vi "rsidr_core_global.vi"() -> ()   [LabVIEW 2015, in "Rohde&Schwarz CMXP GPRF.lvlib"] (continued)
Callback"="", "Supported Models"="", "Instrument Options"="", "Flags"=0, "Help"="Returns the traces of the spectrum diagram. The current, average, minimum and maximum traces can be retrieved.\nEach trace contains 801 power values and covers the configured frequency span.\n\nAvailable Repeated Capabilities:\ninstance: i0, i1, i2, i3, i4, i5, i6, i7, i8, i9, i10, i11, i12, i13, i14, i15, i16, i17, i18, i19, i20, i21, i22, i23, i24, i25, i26, i27, i28, i29, i30, i31, i32\r\n\nRemote-control command(s):\nFETCh:GPRF:MEAS<i>:FFTSanalyzer:POWer:MINimum?"}, {"Level"=3, "Class Only"=FALSE, "Identifier"="RSCMXPGPRF_ATTR_FETCH_FFT_MEASUREMENT_POWER_MAXIMUM", "Descriptive Name"="Fetch FFT Measurement Power Maximum", "Data Type"=6, "Command"="FETC:GPRF:MEAS{instance}:FFTS:POW:MAX?", "Access"=0, "Range Table"="", "Read Callback"="", "Write Callback"="", "Supported Models"="", "Instrument Options"="", "Flags"=0, "Help"="Returns the traces of the spectrum diagram. The current, average, minimum and maximum traces can be retrieved.\nEach trace contains 801 power values and covers the configured frequency span.\n\nAvailable Repeated Capabilities:\ninstance: i0, i1, i2, i3, i4, i5, i6, i7, i8, i9, i10, i11, i12, i13, i14, i15, i16, i17, i18, i19, i20, i21, i22, i23, i24, i25, i26, i27, i28, i29, i30, i31, i32\r\n\nRemote-control command(s):\nFETCh:GPRF:MEAS<i>:FFTSanalyzer:POWer:MAXimum?"}, {"Level"=3, "Class Only"=FALSE, "Identifier"="RSCMXPGPRF_ATTR_READ_FFT_MEASUREMENT_PEAK_SEARCH_RESULT_CURRENT", "Descriptive Name"="Read FFT Measurement Peak Search Result Current", "Data Type"=6, "Command"="READ:GPRF:MEAS{instance}:FFTS:PEAK:CURR?", "Access"=0, "Range Table"="", "Read Callback"="", "Write Callback"="", "Supported Models"="", "Instrument Options"="", "Flags"=0, "Help"="Returns the results of the peak search in the spectrum diagram. Separate commands retrieve results for the current trace and for the average trace.\nThe results are returned in the following order:\n<Reliability>, {<Frequency>, <Level>}marker 0, ..., {<Frequency>, <Level>}marker 4\n\nAvailable Repeated Capabilities:\ninstance: i0, i1, i2, i3, i4, i5, i6, i7, i8, i9, i10, i11, i12, i13, i14, i15, i16, i17, i18, i19, i20, i21, i22, i23, i24, i25, i26, i27, i28, i29, i30, i31, i32\r\n\nRemote-control command(s):\nREAD:GPRF:MEAS<i>:FFTSanalyzer:PEAKs:CURRent?"}, {"Level"=3, "Class Only"=FALSE, "Identifier"="RSCMXPGPRF_ATTR_READ_FFT_MEASUREMENT_PEAK_SEARCH_RESULT_AVERAGE", "Descriptive Name"="Read FFT Measurement Peak Search Result Average", "Data Type"=6, "Command"="READ:GPRF:MEAS{instance}:FFTS:PEAK:AVER?", "Access"=0, "Range Table"="", "Read Callback"="", "Write Callback"="", "Supported Models"="", "Instrument Options"="", "Flags"=0, "Help"="Returns the results of the peak search in the spectrum diagram. Separate commands retrieve results for the current trace and for the average trace.\nThe results are returned in the following order:\n<Reliability>, {<Frequency>, <Level>}marker 0, ..., {<Frequency>, <Level>}marker 4\n\nAvailable Repeated Capabilities:\ninstance: i0, i1, i2, i3, i4, i5, i6, i7, i8, i9, i10, i11, i12, i13, i14, i15, i16, i17, i18, i19, i20, i21, i22, i23, i24, i25, i26, i27, i28, i29, i30, i31, i32\r\n\nRemote-control command(s):\nREAD:GPRF:MEAS<i>:FFTSanalyzer:PEAKs:AVERage?"}, {"Level"=3, "Class Only"=FALSE, "Identifier"="RSCMXPGPRF_ATTR_FETCH_FFT_MEASUREMENT_PEAK_SEARCH_RESULT_CURRENT", "Descriptive Name"="Fetch FFT Measurement Peak Search Result Current", "Data Type"=6, "Command"="FETC:GPRF:MEAS{instance}:FFTS:PEAK:CURR?", "Access"=0, "Range Table"="", "Read Callback"="", "Write Callback"="", "Supported Models"="", "Instrument Options"="", "Flags"=0, "Help"="Returns the results of the peak search in the spectrum diagram. Separate commands retrieve results for the current trace and for the average trace.\nThe results are returned in the following order:\n<Reliability>, {<Frequency>, <Level>}marker 0, ..., {<Frequency>, <Level>}marker 4\n\nAvailable Repeated Capabilities:\ninstance: i0, i1, i2, i3, i4, i5, i6, i7, i8, i9, i10, i11, i12, i13, i14, i15, i16, i17, i18, i19, i20, i21, i22, i23, i24, i25, i26, i27, i28, i29, i30, i31, i32\r\n\nRemote-control command(s):\nFETCh:GPRF:MEAS<i>:FFTSanalyzer:PEAKs:CURRent?"}, {"Level"=3, "Class Only"=FALSE, "Identifier"="RSCMXPGPRF_ATTR_FETCH_FFT_MEASUREMENT_PEAK_SEARCH_RESULT_AVERAGE", "Descriptive Name"="Fetch FFT Measurement Peak Search Result Average", "Data Type"=6, "Command"="FETC:GPRF:MEAS{instance}:FFTS:PEAK:AVER?", "Access"=0, "Range Table"="", "Read Callback"="", "Write Callback"="", "Supported Models"="", "Instrument Options"="", "Flags"=0, "Help"="Returns the results of the peak search in the spectrum diagram. Separate commands retrieve results for the current trace and for the average trace.\nThe results are returned in the following order:\n<Reliability>, {<Frequency>, <Level>}marker 0, ..., {<Frequency>, <Level>}marker 4\n\nAvailable Repeated Capabilities:\ninstance: i0, i1, i2, i3, i4, i5, i6, i7, i8, i9, i10, i11, i12, i13, i14, i15, i16, i17, i18, i19, i20, i21, i22, i23, i24, i25, i26, i27, i28, i29, i30, i31, i32\r\n\nRemote-control command(s):\nFETCh:GPRF:MEAS<i>:FFTSanalyzer:PEAKs:AVERage?"}, {"Level"=3, "Class Only"=FALSE, "Identifier"="RSCMXPGPRF_ATTR_READ_FFT_MEASUREMENT_IQ_AMPLITUDES_I", "Descriptive Name"="Read FFT Measurement IQ Amplitudes I", "Data Type"=6, "Command"="READ:GPRF:MEAS{instance}:FFTS:I?", "Access"=0, "Range Table"="", "Read Callback"="", "Write Callback"="", "Supported Models"="", "Instrument Options"="", "Flags"=0, "Help"="Returns the measured normalized I and Q amplitudes in the time domain.\n\nAvailable Repeated Capabilities:\ninstance: i0, i1, i2, i3, i4, i5, i6, i7, i8, i9, i10, i11, i12, i13, i14, i15, i16, i17, i18, i19, i20, i21, i22, i23, i24, i25, i26, i27, i28, i29, i30, i31, i32\r\n\nRemote-control command(s):\nREAD:GPRF:MEAS<i>:FFTSanalyzer:I?"}, {"Level"=3, "Class Only"=FALSE, "Identifier"="RSCMXPGPRF_ATTR_READ_FFT_MEASUREMENT_IQ_AMPLITUDES_Q", "Descriptive Name"="Read FFT Measurement IQ Amplitudes Q", "Data Type"=6, "Command"="READ:GPRF:MEAS{instance}:FFTS:Q?", "Access"=0, "Range Table"="", "Read Callback"="", "Write Callback"="", "Supported Models"="", "Instrument Options"="", "Flags"=0, "Help"="Returns the measured normalized I and Q amplitudes in the time domain.\n\nAvailable Repeated Capabilities:\ninstance: i0, i1, i2, i3, i4, i5, i6, i7, i8, i9, i10, i11, i12, i13, i14, i15, i16, i17, i18, i19, i20, i21, i22, i23, i24, i25, i26, i27, i28, i29, i30, i31, i32\r\n\nRemote-control command(s):\nREAD:GPRF:MEAS<i>:FFTSanalyzer:Q?"}, {"Level"=3, "Class Only"=FALSE, "Identifier"="RSCMXPGPRF_ATTR_FETCH_FFT_MEASUREMENT_IQ_AMPLITUDES_I", "Descriptive Name"="Fetch FFT Measurement IQ Amplitudes I", "Data Type"=6, "Command"="FETC:GPRF:MEAS{instance}:FFTS:I?", "Access"=0, "Range Table"="", "Read Callback"="", "Write Callback"="", "Supported Models"="", "Instrument Options"="", "Flags"=0, "Help"="Returns the measured normalized I and Q amplitudes in the time domain.\n\nAvailable Repeated Capabilities:\ninstance: i0, i1, i2, i3, i4, i5, i6, i7, i8, i9, i10, i11, i12, i13, i14, i15, i16, i17, i18, i19, i20, i21, i22, i23, i24, i25, i26, i27, i28, i29, i30, i31, i32\r\n\nRemote-control command(s):\nFETCh:GPRF:MEAS<i>:FFTSanalyzer:I?"}, {"Level"=3, "Class Only"=FALSE, "Identifier"="RSCMXPGPRF_ATTR_FETCH_FFT_MEASUREMENT_IQ_AMPLITUDES_Q", "Descriptive Name"="Fetch FFT Measurement IQ Amplitudes Q", "Data Type"=6, "Command"="FETC:GPRF:MEAS{instance}:FFTS:Q?", "Access"=0, "Range Table"="", "Read Callback"="", "Write Callback"="", "Supported Models"="", "Instrument Options"="", "Flags"=0, "Help"="Returns the measured normalized I and Q amplitudes in the time domain.\n\nAvailable Repeated Capabilities:\ninstance: i0, i1, i2, i3, i4, i5, i6, i7, i8, i9, i10, i11, i12, i13, i14, i15, i16, i17, i18, i19, i20, i21, i22, i23, i24, i25, i26, i27, i28, i29, i30, i31, i32\r\n\nRemote-control command(s):\nFETCh:GPRF:MEAS<i>:FFTSanalyzer:Q?"}, {"Level"=1, "Class Only"=TRUE, "Identifier"="", "Descriptive Name"="Capture Analyzer", "Data Type"=0, "Command"="", "Access"=0, "Range Table"="", "Read Callback"="", "Write Callback"="", "Supported Models"="", "Instrument Options"="", "Flags"=0, "Help"="Configures the Capture Analyzer Square."}, {"Level"=2, "Class Only"=TRUE, "Identifier"="", "Descriptive Name"="Configuration", "Data Type"=0, "Command"="", "Access"=0, "Range Table"="", "Read Callback"="", "Write Callback"="", "Supported Models"="", "Instrument Options"="", "Flags"=0, "Help"="Configures the Capture Analyzer Square."}, {"Level"=3, "Class Only"=FALSE, "Identifier"="RSCMXPGPRF_ATTR_CAPTURE_ANALYZER_MEASUREMENT_SEGMENT", "Descriptive Name"="Capture Analyzer Measurement Segment", "Data Type"=0, "Command"="CONF:GPRF:MEAS{instance}:CAN:SEGM", "Access"=2, "Range Table"="", "Read Callback"="", "Write Callback"="", "Supported Models"="", "Instrument Options"="", "Flags"=0, "Help"="Selects a segment of a list mode measurement for result analysis.\nThe selection affects the GUI contents and the contents stored by the command CONFigure:GPRF:MEAS<i>:CANalyzer:IQFile.\n\nAvailable Repeated Capabilities:\ninstance: i0, i1, i2, i3, i4, i5, i6, i7, i8, i9, i10, i11, i12, i13, i14, i15, i16, i17, i18, i19, i20, i21, i22, i23, i24, i25, i26, i27, i28, i29, i30, i31, i32\r\n\nRemote-control command(s):\nCONFigure:GPRF:MEAS<i>:CANalyzer:SEGMent"}, {"Level"=3, "Class Only"=FALSE, "Identifier"="RSCMXPGPRF_ATTR_CAPTURE_ANALYZER_MEASUREMENT_STEP", "Descriptive Name"="Capture Analyzer Measurement Step", "Data Type"=0, "Command"="CONF:GPRF:MEAS{instance}:CAN:STEP", "Access"=2, "Range Table"="", "Read Callback"="", "Write Callback"="", "Supported Models"="", "Instrument Options"="", "Flags"=0, "Help"="Selects a step of a list mode measurement for result analysis.\nThe selection affects the GUI contents and the contents stored by the command CONFigure:GPRF:MEAS<i>:CANalyzer:IQFile.\n\nAvailable Repeated Capabilities:\ninstance: i0, i1, i2, i3, i4, i5, i6, i7, i8, i9, i10, i11, i12, i13, i14, i15, i16, i17, i18, i19, i20, i21, i22, i23, i24, i25, i26, i27, i28, i29, i30, i31, i32\r\n\nRemote-control command(s):\nCONFigure:GPRF:MEAS<i>:CANalyzer:STEP"}, {"Level"=3, "Class Only"=FALSE, "Identifier"="RSCMXPGPRF_ATTR_CAPTURE_ANALYZER_MEASUREMENT_SAVE_IQ_FILE", "Descriptive Name"="Capture Analyzer Measurement Save IQ File", "Data Type"=2, "Command"="CONF:GPRF:MEAS{instance}:CAN:IQF", "Access"=2, "Range Table"="", "Read Callback"="", "Write Callback"="", "Supported Models"="", "Instrument Options"="", "Flags"=0, "Help"="Saves the I/Q data for the current step to the selected file.\n\nAvailable Repeated Capabilities:\ninstance: i0, i1, i2, i3, i4, i5, i6, i7, i8, i9, i10, i11, i12, i13, i14, i15, i16, i17, i18, i19, i20, i21, i22, i23, i24, i25, i26, i27, i28, i29, i30, i31, i32\r\n\nRemote-control command(s):\nCONFigure:GPRF:MEAS<i>:CANalyzer:IQFile"}, {"Level"=3, "Class Only"=FALSE, "Identifier"="RSCMXPGPRF_ATTR_CAPTURE_ANALYZER_MEASUREMENT_STORAGE_FOLDER", "Descriptive Name"="Capture Analyzer Measurement Storage Folder", "Data Type"=2, "Command"="CONF:GPRF:MEAS{instance}:CAN:SALL:IQF", "Access"=2, "Range Table"="", "Read Callback"="", "Write Callback"="", "Supported Models"="", "Instrument Options"="", "Flags"=0, "Help"="Selects a folder for storage of all buffer contents to files (I/Q data for all segments).\nThe default folder is @USERDATA\\captureanalyzer. You can only select a subfolder of this default folder.\nAll files within the selected folder are deleted when the capture buffer analyzer writes the result files.\n\nAvailable Repeated Capabilities:\ninstance: i0, i1, i2, i3, i4, i5, i6, i7, i8, i9, i10, i11, i12, i13, i14, i15, i16, i17, i18, i19, i20, i21, i22, i23, i24, i25, i26, i27, i28, i29, i30, i31, i32\r\n\nRemote-control command(s):\nCONFigure:GPRF:MEAS<i>:CANalyzer:SALL:IQFolder"}, {"Level"=3, "Class Only"=FALSE, "Identifier"="RSCMXPGPRF_ATTR_CAPTURE_ANALYZER_MEASUREMENT_WRITE_TO_FILE", "Descriptive Name"="Capture Analyzer Measurement Write to File", "Data Type"=3, "Command"="CONF:GPRF:MEAS{instance}:CAN:SALL:WTF", "Access"=2, "Range Table"="", "Read Callback"="", "Write Callback"="", "Supported Models"="", "Instrument Options"="", "Flags"=0, "Help"="Enables or disables saving of all buffer contents to files (I/Q data for all segments).\nWith <WriteToFolder> = ON, the files are stored when the capture buffer analyzer is started.\n\nAvailable Repeated Capabilities:\ninstance: i0, i1, i2, i3, i4, i5, i6, i7, i8, i9, i10, i11, i12, i13, i14, i15, i16, i17, i18, i19, i20, i21, i22, i23, i24, i25, i26, i27, i28, i29, i30, i31, i32\r\n\nRemote-control command(s):\nCONFigure:GPRF:MEAS<i>:CANalyzer:SALL:WTFolder"}, {"Level"=2, "Class Only"=TRUE, "Identifier"="", "Descriptive Name"="Control", "Data Type"=0, "Command"="", "Access"=0, "Range Table"="", "Read Callback"="", "Write Callback"="", "Supported Models"="", "Instrument Options"="", "Flags"=0, "Help"="Configures the Capture Analyzer Square Control."}, {"Level"=3, "Class Only"=FALSE, "Identifier"="RSCMXPGPRF_ATTR_CAPTURE_ANALYZER_MEASUREMENT_INIT", "Descriptive Name"="Capture Analyzer Measurement Init", "Data Type"=4, "Command"="INIT:GPRF:MEAS{instance}:CAN", "Access"=1, "Range Table"="", "Read Callback"="", "Write Callback"="", "Supported Models"="", "Instrument Options"="", "Flags"=0, "Help"="Starts the measurement.\n\nAvailable Repeated Capabilities:\ninstance: i0, i1, i2, i3, i4, i5, i6, i7, i8, i9, i10, i11, i12, i13, i14, i15, i16, i17, i18, i19, i20, i21, i22, i23, i24, i25, i26, i27, i28, i29, i30, i31, i32\r\n\nRemote-control command(s):\nINITiate:GPRF:MEAS<i>:CANalyzer"}, {"Level"=3, "Class Only"=FALSE, "Identifier"="RSCMXPGPRF_ATTR_CAPTURE_ANALYZER_MEASUREMENT_ABORT", "Descriptive Name"="Capture Analyzer Measurement Abort", "Data Type"=4, "Command"="ABOR:GPRF:MEAS{instance}:CAN", "Access"=1, "Range Table"="", "Read Callback"="", "Write Callback"="", "Supported Models"="", "Instrument Options"="", "Flags"=0, "Help"="Aborts the measurement.\n\nAvailable Repeated Capabilities:\ninstance: i0, i1, i2, i3, i4, i5, i6, i7, i8, i9, i10, i11, i12, i13, i14, i15, i16, i17, i18, i19, i20, i21, i22, i23, i24, i25, i26, i27, i28, i29, i30, i31, i32\r\n\nRemote-control command(s):\nABORt:GPRF:MEAS<i>:CANalyzer"}, {"Level"=3, "Class Only"=FALSE, "Identifier"="RSCMXPGPRF_ATTR_CAPTURE_ANALYZER_MEASUREMENT_STOP", "Descriptive Name"="Capture Analyzer Measurement Stop", "Data Type"=4, "Command"="STOP:GPRF:MEAS{instance}:CAN", "Access"=1, "Range Table"="", "Read Callback"="", "Write Callback"="", "Supported Models"="", "Instrument Options"="", "Flags"=0, "Help"="Stops the measurement.\n\nAvailable Repeated Capabilities:\ninstance: i0, i1, i2, i3, i4, i5, i6, i7, i8, i9, i10, i11, i12, i13, i14, i15, i16, i17, i18, i19, i20, i21, i22, i23, i24, i25, i26, i27, i28, i29, i30, i31, i32\r\n\nRemote-control command(s):\nSTOP:GPRF:MEAS<i>:CANalyzer"}, {"Level"=3, "Class Only"=FALSE, "Identifier"="RSCMXPGPRF_ATTR_CAPTURE_ANALYZER_MEASUREMENT_STATUS", "Descriptive Name"="Capture Analyzer Measurement Status", "Data Type"=6, "Command"="FETC:GPRF:MEAS{instance}:CAN:STAT?", "Access"=0, "Range Table"="", "Read Callback"="", "Write Callback"="", "Supported Models"="", "Instrument Options"="", "Flags"=0, "Help"="Queries the main measurement state.\n\nAvailable Repeated Capabilities:\ninstance: i0, i1, i2, i3, i4, i5, i6, i7, i8, i9, i10, i11, i12, i13, i14, i15, i16, i17, i18, i19, i20, i21, i22, i23, i24, i25, i26, i27, i28, i29, i30, i31, i32\r\n\nRemote-control command(s):\nFETCh:GPRF:MEAS<i>:CANalyzer:STATe?"}, {"Level"=3, "Class Only"=FALSE, "Identifier"="RSCMXPGPRF_ATTR_CAPTURE_ANALYZER_MEASUREMENT_STATUS_ALL", "Descriptive Name"="Capture Analyzer Measurement Status All", "Data Type"=6, "Command"="FETC:GPRF:MEAS{instance}:CAN:STAT:ALL?", "Access"=0, "Range Table"="", "Read Callback"="", "Write Callback"="", "Supported Models"="", "Instrument Options"="", "Flags"=0, "Help"="Queries the main measurement state and the measurement substates. Both measurement substates are relevant for running measurements only.\n\nAvailable Repeated Capabilities:\ninstance: i0, i1, i2, i3, i4, i5, i6, i7, i8, i9, i10, i11, i12, i13, i14, i15, i16, i17, i18, i19, i20, i21, i22, i23, i24, i25, i26, i27, i28, i29, i30, i31, i32\r\n\nRemote-control command(s):\nFETCh:GPRF:MEAS<i>:CANalyzer:STATe:ALL?"}, {"Level"=3, "Class Only"=FALSE, "Identifier"="RSCMXPGPRF_ATTR_CAPTURE_ANALYZER_MEASUREMENT_FIRMWARE", "Descriptive Name"="Capture Analyzer Measurement Firmware", "Data Type"=2, "Command"="CONF:GPRF:MEAS{instance}:CAN:MNAM?", "Access"=0, "Range Table"="", "Read Callback"="", "Write Callback"="", "Supported Models"="", "Instrument Options"="", "Flags"=0, "Help"="Queries which firmware application has captured the data.\n\nAvailable Repeated Capabilities:\ninstance: i0, i1, i2, i3, i4, i5, i6, i7, i8, i9, i10, i11, i12, i13, i14, i15, i16, i17, i18, i19, i20, i21, i22, i23, i24, i25, i26, i27, i28, i29, i30, i31, i32\r\n\nRemote-control command(s):\nCONFigure:GPRF:MEAS<i>:CANalyzer:MNAMe?"}, {"Level"=1, "Class Only"=TRUE, "Identifier"="", "Descriptive Name"="NRPM", "Data Type"=0, "Command"="", "Access"=0, "Range Table"="", "Read Callback"="", "Write Callback"="", "Supported Models"="", "Instrument Options"="", "Flags"=0, "Help"="Configures the NRPM Square."}, {"Level"=2, "Class Only"=TRUE, "Identifier"="", "Descriptive Name"="Configuration", "Data Type"=0, "Command"="", "Access"=0, "Range Table"="", "Read Callback"="", "Write Callback"="", "Supported Models"="", "Instrument Options"="", "Flags"=0, "Help"="Configures the NRPM Square."}, {"Level"=3, "Class Only"=FALSE, "Identifier"="RSCMXPGPRF_ATTR_NRPM_MEASUREMENT_FREQUENCY", "Descriptive Name"="NRPM Measurement Frequency", "Data Type"=1, "Command"="CONF:GPRF:MEAS{instance}:NRPM:SENS{sensor}:FREQ", "Access"=2, "Range Table"="rsCmxpGprf_rngNRPMMeasurementFrequency", "Read Callback"="", "Write Callback"="", "Supported Models"="", "Instrument Options"="", "Flags"=0, "Help"="Specifies the input frequency at the power sensor connected to Sensor.\n\nAvailable Repeated Capabilities:\ninstance: i0, i1, i2, i3, i4, i5, i6, i7, i8, i9, i10, i11, i12, i13, i14, i15, i16, i17, i18, i19, i20, i21, i22, i23, i24, i25, i26, i27, i28, i29, i30, i31, i32\r\nsensor: sensor1, sensor2, sensor3\r\n\nRemote-control command(s):\nCONFigure:GPRF:MEAS<i>:NRPM:SENSor<no>:FREQuency"}, {"Level"=3, "Class Only"=FALSE, "Identifier"="RSCMXPGPRF_ATTR_NRPM_MEASUREMENT_TIMEOUT", "Descriptive Name"="NRPM Measurement Timeout", "Data Type"=1, "Command"="CONF:GPRF:MEAS{instance}:NRPM:TOUT", "Access"=2, "Range Table"="", "Read Callback"="", "Write Callback"="", "Supported Models"="", "Instrument Options"="", "Flags"=0, "Help"="Defines a timeout for the measurement. The timer is started when the measurement is initiated via a READ or INIT command. It is not started if the measurement is initiated manually ([ON | OFF] key or [RESTART | STOP] key).When the measurement has completed the first measurement cycle (first single shot), the statistical depth is reached and the timer is reset.If the first measurement cycle has not been completed when the timer expires, the measurement is stopped. The measurement state  changes to RDY. The reliability indicator is set to 1, indicating that a measurement timeout occurred. Still running READ, FETCh or CALCulate commands are completed, returning the available results. At least for some results, there are no values at all or the statistical depth has not been reached.A timeout of 0 s corresponds to an infinite measurement timeout.\n\nAvailable Repeated Capabilities:\ninstance: i0, i1, i2, i3, i4, i5, i6, i7, i8, i9, i10, i11, i12, i13, i14, i15, i16, i17, i18, i19, i20, i21, i22, i23, i24, i25, i26, i27, i28, i29, i30, i31, i32\r\n\nRemote-control command(s):\nCONFigure:GPRF:MEAS<i>:NRPM:TOUT"}, {"Level"=3, "Class Only"=FALSE, "Identifier"="RSCMXPGPRF_ATTR_NRPM_MEASUREMENT_STATISTIC_COUNT", "Descriptive Name"="NRPM Measurement Statistic Count", "Data Type"=0, "Command"="CONF:GPRF:MEAS{instance}:NRPM:SCO", "Access"=2, "Range Table"="rsCmxpGprf_rngNRPMStatCount", "Read Callback"="", "Write Callback"="", "Supported Models"="", "Instrument Options"="", "Flags"=0, "Help"="Specifies the statistic count of the measurement. The statistic count is equal to the number of measurement intervals per single shot.\n\nAvailable Repeated Capabilities:\ninstance: i0, i1, i2, i3, i4, i5, i6, i7, i8, i9, i10, i11, i12, i13, i14, i15, i16, i17, i18, i19, i20, i21, i22, i23, i24, i25, i26, i27, i28, i29, i30, i31, i32\r\n\nRemote-control command(s):\nCONFigure:GPRF:MEAS<i>:NRPM:SCOunt"}, {"Level"=3, "Class Only"=FALSE, "Identifier"="RSCMXPGPRF_ATTR_NRPM_MEASUREMENT_REPETITION", "Descriptive Name"="NRPM Measurement Repetition", "Data Type"=0, "Command"="CONF:GPRF:MEAS{instance}:NRPM:REP", "Access"=2, "Range Table"="rsCmxpGprf_rngRepMode", "Read Callback"="", "Write Callback"="", "Supported Models"="", "Instrument Options"="", "Flags"=0, "Help"="Specifies the repetition mode of the measurement. The repetition mode specifies whether the measurement is stopped after a single shot or repeated continuously. Use CONFigure:..:MEAS<i>:...:SCOunt to determine the number of measurement intervals per single shot.\n\nAvailable Repeated Capabilities:\ninstance: i0, i1, i2, i3, i4, i5, i6, i7, i8, i9, i10, i11, i12, i13, i14, i15, i16, i17, i18, i19, i20, i21, i22, i23, i24, i25, i26, i27, i28, i29, i30, i31, i32\r\n\nRemote-control command(s):\nCONFigure:GPRF:MEAS<i>:NRPM:REPetition"}, {"Level"=2, "Class Only"=TRUE, "Identifier"="", "Descriptive Name"="Control", "Data Type"=0, "Command"="", "Access"=0, "Range Table"="", "Read Callback"="", "Write Callback"="", "Supported Models"="", "Instrument Options"="", "Flags"=0, "Help"="Configures the NRPM Square Control."}, {"Level"=3, "Class Only"=FALSE, "Identifier"="RSCMXPGPRF_ATTR_NRPM_MEASUREMENT_INIT", "Descriptive Name"="NRPM Measurement Init", "Data Type"=4, "Command"="INIT:GPRF:MEAS{instance}:NRPM", "Access"=1, "Range Table"="", "Read Callback"="", "Write Callback"="", "Supported Models"="", "Instrument Options"="", "Flags"=0, "Help"="Starts the measurement.\n\nAvailable Repeated Capabilities:\ninstance: i0, i1, i2, i3, i4, i5, i6, i7, i8, i9, i10, i11, i12, i13, i14, i15, i16, i17, i18, i19, i20, i21, i22, i23, i24, i25, i26, i27, i28, i29, i30, i31, i32\r\n\nRemote-control command(s):\nINITiate:GPRF:MEAS<i>:NRPM"}, {"Level"=3, "Class Only"=FALSE, "Identifier"="RSCMXPGPRF_ATTR_NRPM_MEASUREMENT_ABORT", "Descriptive Name"="NRPM Measurement Abort", "Data Type"=4, "Command"="ABOR:GPRF:MEAS{instance}:NRPM", "Access"=1, "Range Table"="", "Read Callback"="", "Write Callback"="", "Supported Models"="", "Instrument Options"="", "Flags"=0, "Help"="Aborts the measurement.\n\nAvailable Repeated Capabilities:\ninstance: i0, i1, i2, i3, i4, i5, i6, i7, i8, i9, i10, i11, i12, i13, i14, i15, i16, i17, i18, i19, i20, i21, i22, i23, i24, i25, i26, i27, i28, i29, i30, i31, i32\r\n\nRemote-control command(s):\nABORt:GPRF:MEAS<i>:NRPM"}, {"Level"=3, "Class Only"=FALSE, "Identifier"="RSCMXPGPRF_ATTR_NRPM_MEASUREMENT_STOP", "Descriptive Name"="NRPM Measurement Stop", "Data Type"=4, "Command"="STOP:GPRF:MEAS{instance}:NRPM", "Access"=1, "Range Table"="", "Read Callback"="", "Write Callback"="", "Supported Models"="", "Instrument Options"="", "Flags"=0, "Help"="Stops the measurement.\n\nAvailable Repeated Capabilities:\ninstance: i0, i1, i2, i3, i4, i5, i6, i7, i8, i9, i10, i11, i12, i13, i14, i15, i16, i17, i18, i19, i20, i21, i22, i23, i24, i25, i26, i27, i28, i29, i30, i31, i32\r\n\nRemote-control command(s):\nSTOP:GPRF:MEAS<i>:NRPM"}, {"Level"=3, "Class Only"=FALSE, "Identifier"="RSCMXPGPRF_ATTR_NRPM_MEASUREMENT_STATUS", "Descriptive Name"="NRPM Measurement Status", "Data Type"=6, "Command"="FETC:GPRF:MEAS{instance}:NRPM:STAT?", "Access"=0, "Range Table"="", "Read Callback"="", "Write Callback"="", "Supported Models"="", "Instrument Options"="", "Flags"=0, "Help"="Queries the main measurement state.\n\nAvailable Repeated Capabilities:\ninstance: i0, i1, i2, i3, i4, i5, i6, i7, i8, i9, i10, i11, i12, i13, i14, i15, i16, i17, i18, i19, i20, i21, i22, i23, i24, i25, i26, i27, i28, i29, i30, i31, i32\r\n\nRemote-control command(s):\nFETCh:GPRF:MEAS<i>:NRPM:STATe?"}, {"Level"=3, "Class Only"=FALSE, "Identifier"="RSCMXPGPRF_ATTR_NRPM_MEASUREMENT_STATUS_ALL", "Descriptive Name"="NRPM Measurement Status All", "Data Type"=6, "Command"="FETC:GPRF:MEAS{instance}:NRPM:STAT:ALL?", "Access"=0, "Range Table"="", "Read Callback"="", "Write Callback"="", "Supported Models"="", "Instrument Options"="", "Flags"=0, "Help"="Queries the main measurement state and the measurement substates. Both measurement substates are relevant for running measurements only.\n\nAvailable Repeated Capabilities:\ninstance: i0, i1, i2, i3, i4, i5, i6, i7, i8, i9, i10, i11, i12, i13, i14, i15, i16, i17, i18, i19, i20, i21, i22, i23, i24, i25, i26, i27, i28, i29, i30, i31, i32\r\n\nRemote-control command(s):\nFETCh:GPRF:MEAS<i>:NRPM:STATe:ALL?"}, {"Level"=2, "Class Only"=TRUE, "Identifier"="", "Descriptive Name"="Results", "Data Type"=0, "Command"="", "Access"=0, "Range Table"="", "Read Callback"="", "Write Callback"="", "Supported Models"="", "Instrument Options"="", "Flags"=0, "Help"="Queries the NRPM Square Results."}, {"Level"=3, "Class Only"=FALSE, "Identifier"="RSCMXPGPRF_ATTR_NRPM_MEASUREMENT_SENSOR_POWER", "Descriptive Name"="NRPM Measurement Sensor Power", "Data Type"=6, "Command"="CALC:GPRF:MEAS{instance}:NRPM:SENS{sensor}:POW?", "Access"=0, "Range Table"="", "Read Callback"="", "Write Callback"="", "Supported Models"="", "Instrument Options"="", "Flags"=0, "Help"="Returns the measurement results for the power sensor connected to Sensor <no>.\n\nAvailable Repeated Capabilities:\ninstance: i0, i1, i2, i3, i4, i5, i6, i7, i8, i9, i10, i11, i12, i13, i14, i15, i16, i17, i18, i19, i20, i21, i22, i23, i24, i25, i26, i27, i28, i29, i30, i31, i32\r\nsensor: sensor1, sensor2, sensor3\r\n\nRemote-control command(s):\nCALCulate:GPRF:MEAS<i>:NRPM:SENSor<no>:POWer?"}, {"Level"=3, "Class Only"=FALSE, "Identifier"="RSCMXPGPRF_ATTR_FETCH_NRPM_MEASUREMENT_SENSOR_POWER", "Descriptive Name"="Fetch NRPM Measurement Sensor Power", "Data Type"=6, "Command"="FETC:GPRF:MEAS{instance}:NRPM:SENS{sensor}:POW?", "Access"=0, "Range Table"="", "Read Callback"="", "Write Callback"="", "Supported Models"="", "Instrument Options"="", "Flags"=0, "Help"="Returns the measurement results for the power sensor connected to Sensor <no>.\n\nAvailable Repeated Capabilities:\ninstance: i0, i1, i2, i3, i4, i5, i6, i7, i8, i9, i10, i11, i12, i13, i14, i15, i16, i17, i18, i19, i20, i21, i22, i23, i24, i25, i26, i27, i28, i29, i30, i31, i32\r\nsensor: sensor1, sensor2, sensor3\r\n\nRemote-control command(s):\nFETCh:GPRF:MEAS<i>:NRPM:SENSor<no>:POWer?"}, {"Level"=3, "Class Only"=FALSE, "Identifier"="RSCMXPGPRF_ATTR_READ_NRPM_MEASUREMENT_SENSOR_POWER", "Descriptive Name"="Read NRPM Measurement Sensor Power", "Data Type"=6, "Command"="READ:GPRF:MEAS{instance}:NRPM:SENS{sensor}:POW?", "Access"=0, "Range Table"="", "Read Callback"="", "Write Callback"="", "Supported Models"="", "Instrument Options"="", "Flags"=0, "Help"="Returns the measurement results for the power sensor connected to Sensor <no>.\n\nAvailable Repeated Capabilities:\ninstance: i0, i1, i2, i3, i4, i5, i6, i7, i8, i9, i10, i11, i12, i13, i14, i15, i16, i17, i18, i19, i20, i21, i22, i23, i24, i25, i26, i27, i28, i29, i30, i31, i32\r\nsensor: sensor1, sensor2, sensor3\r\n\nRemote-control command(s):\nREAD:GPRF:MEAS<i>:NRPM:SENSor<no>:POWer?"}, {"Level"=1, "Class Only"=TRUE, "Identifier"="", "Descriptive Name"="Utility", "Data Type"=0, "Command"="", "Access"=0, "Range Table"="", "Read Callback"="", "Write Callback"="", "Supported Models"="", "Instrument Options"="", "Flags"=0, "Help"="Put a help here"}, {"Level"=2, "Class Only"=FALSE, "Identifier"="RSCMXPGPRF_ATTR_SYSTEM_VERSION", "Descriptive Name"="System Version", "Data Type"=2, "Command"="SYST:VERSion?", "Access"=0, "Range Table"="", "Read Callback"="", "Write Callback"="", "Supported Models"="", "Instrument Options"="", "Flags"=0, "Help"="Gets system version.\n\nAvailable Repeated Capabilities:\nNone\n\nRemote-control command(s):\nSYSTem:VERSion?"}, {"Level"=2, "Class Only"=FALSE, "Identifier"="RSCMXPGPRF_ATTR_SYSTEM_ERROR", "Descriptive Name"="System Error", "Data Type"=2, "Command"="SYST:ERRor?", "Access"=0, "Range Table"="", "Read Callback"="", "Write Callback"="", "Supported Models"="", "Instrument Options"="", "Flags"=0, "Help"="This attribute queries the earliest entry in the error queue, and deletes it after the readout.\n\nAvailable Repeated Capabilities:\nNone\n\nRemote-control command(s):\nSYSTem:ERRor?"}, {"Level"=2, "Class Only"=FALSE, "Identifier"="RSCMXPGPRF_ATTR_SYSTEM_ALL_ERRORS", "Descriptive Name"="System All Errors", "Data Type"=2, "Command"="SYST:ERR:ALL?", "Access"=0, "Range Table"="", "Read Callback"="", "Write Callback"="", "Supported Models"="", "Instrument Options"="", "Flags"=0, "Help"="Reads all errors from instrument.\n\nAvailable Repeated Capabilities:\nNone\n\nRemote-control command(s):\nSYSTem:ERRor:ALL?"}, {"Level"=2, "Class Only"=FALSE, "Identifier"="RSCMXPGPRF_ATTR_SYSTEM_PRESET", "Descriptive Name"="System Preset", "Data Type"=4, "Command"="SYST:PRES", "Access"=1, "Range Table"="", "Read Callback"="", "Write Callback"="", "Supported Models"="", "Instrument Options"="", "Flags"=0, "Help"="Resets instrument.\n\nAvailable Repeated Capabilities:\nNone\n\nRemote-control command(s):\nSYSTem:PRESet"}] {"Flags" format="%08b"; "Access" items=["Read Only", "Write Only", "Read/Write"]; "Data Type" items=["Integer 32", "Double", "String", "Boolean", "None", "Integer 64", "RawString"]}
  in  "Supported Models":string[](array[string])=["CMX", "CMP", "CMW"]
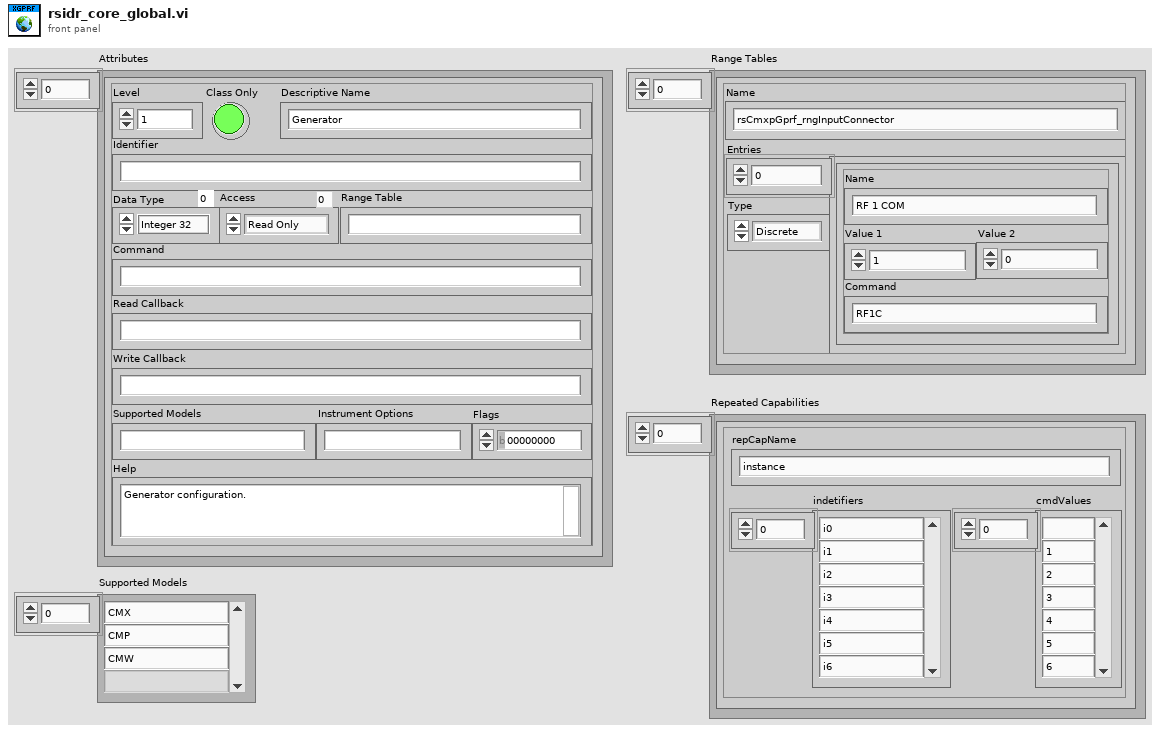
[diagram p1: front panel]
types:
  T1 = typedef "Rohde&Schwarz CMXP GPRF.lvlib/rsidr_core.lvlib/type_Input_Format_RepCap.ctl" = cluster{"repCapName":string, "indetifiers":string[], "cmdValues":string[]}
  T2 = typedef "Rohde&Schwarz CMXP GPRF.lvlib/rsidr_core.lvlib/type_Input_Format_RangeTable.ctl" = cluster{"Type":u16, "Name":string, "Entries":cluster{"Name":string, "Value 1":dbl, "Value 2":dbl, "Command":string}[]}
  T3 = typedef "Rohde&Schwarz CMXP GPRF.lvlib/rsidr_core.lvlib/type_Input_Format_Attribute.ctl" = cluster{"Level":i32, "Class Only":bool, "Identifier":string, "Descriptive Name":string, "Data Type":u16, "Command":string, "Access":u16, "Range Table":string, "Read Callback":string, "Write Callback":string, "Supported Models":string, "Instrument Options":string, "Flags":i32, "Help":string}
diagram:
